vi "WAMP to LV error.vi"(8 "error in (no error)":errorcluster, 9 "Details Index":u32=3, 11 "WAMP Message":T2 {"Message Codes" items=["HELLO"=1, "WELCOME"=2, "ABORT"=3, "GOODBYE"=6, "ERROR"=8, "PUBLISH"=16, "PUBLISHED"=17, "SUBSCRIBE"=32, "SUBSCRIBED"=33, "UNSUBSCRIBE"=34, "UNSUBSCRIBED"=35, "EVENT"=36, "CALL"=48, "RESULT"=59, "REGISTER"=64, "REGISTERED"=65, "UNREGISTER"=66, "UNREGISTERED"=67, "INVOCATION"=68, "YIELD"=70]}) -> (0 "error out":errorcluster, 1 "Cluster":T1={"Details"="{}", "ArgumentKw Payload"="{}", "Error?"=FALSE, "Error URI"="", "Arguments Payload"=[]})   [LabVIEW 2020, in "wamplv.lvlib" / "WAMP Client.lvclass"]
uses:
  <userlib>/wamplv/WAMP Client/WAMP Client.lvclass
  <userlib>/wamplv/WAMP Client/TypeDef/WAMP Received Message.ctl
  <userlib>/wamplv/WAMP Message Codes.ctl
  <userlib>/wamplv/WAMP Client/TypeDef/WAMP Error Payload.ctl
  <vilib>/Utility/error.llb/Error Cluster From Error Code.vi
  <vilib>/ErrorRing/Error Ring.xnode
  <vilib>/JDP Science/JSONtext/JSONtext.lvlib
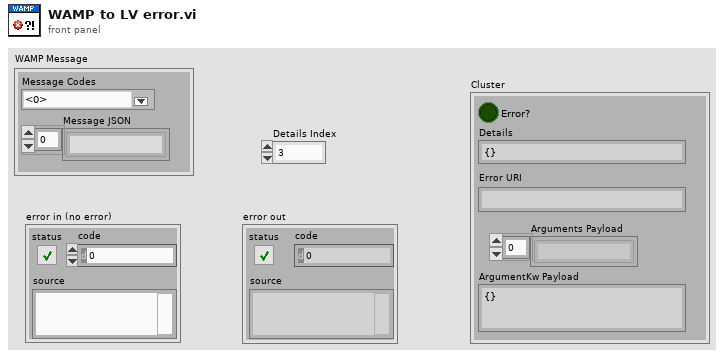
[diagram p1: front panel]
types:
  T1 = typedef "wamplv.lvlib/WAMP Client.lvclass/WAMP Error Payload.ctl" = cluster{"Details":string, "ArgumentKw Payload":string, "Error?":bool, "Error URI":string, "Arguments Payload":string[]}
  T2 = typedef "wamplv.lvlib/WAMP Client.lvclass/WAMP Received Message.ctl" = cluster{"Message JSON":string[], "Message Codes":T3}
  T3 = typedef "wamplv.lvlib/WAMP Client.lvclass/WAMP Message Codes.ctl" = u16
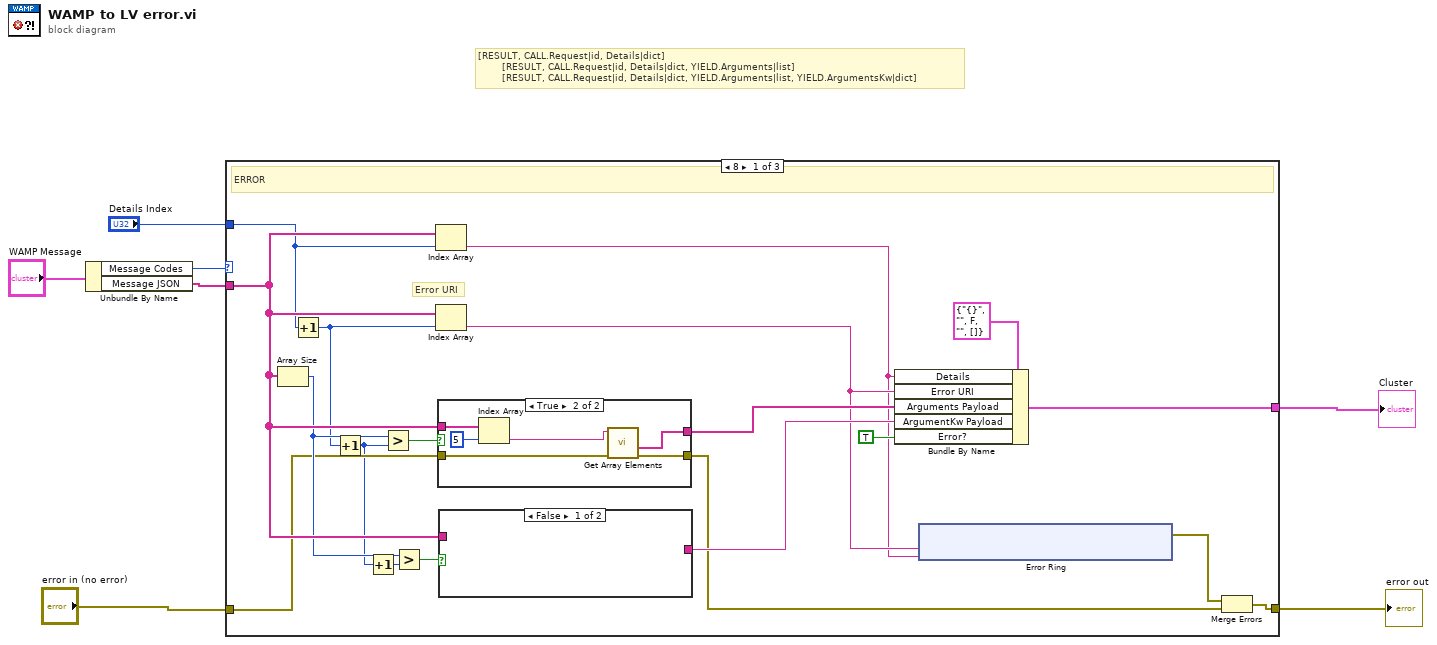
[diagram p0: block diagram]
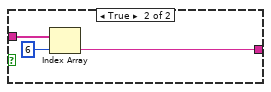
[diagram p2: hidden frame]
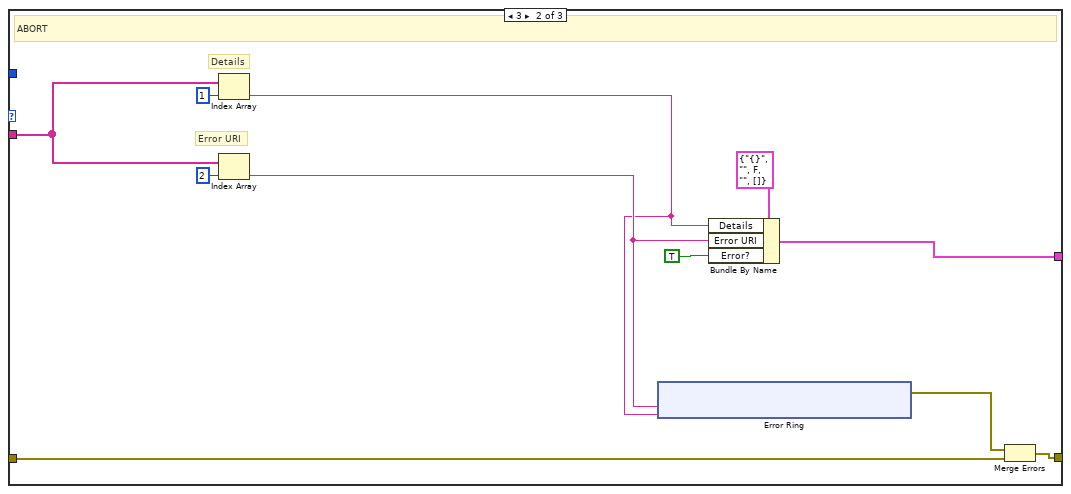
[diagram p4: hidden frame]
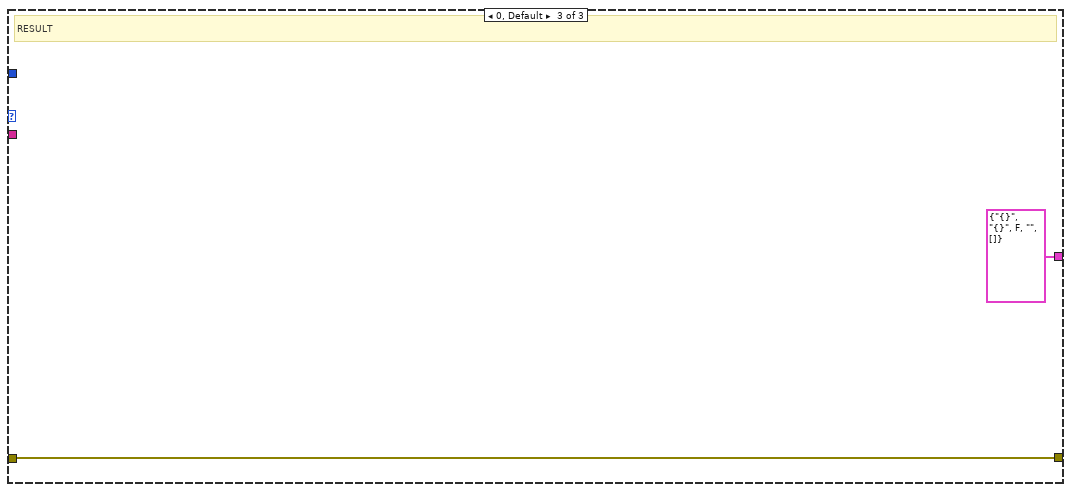
[diagram p5: hidden frame]
diagram:
  # "[RESULT, CALL.Request|id, Details|dict]\n        [RESULT, CALL.Request|id, Details|dict, YIELD.Arguments|list]\n        [RESULT, CALL.Request|id, Details|dict, YIELD.Arguments|list, YIELD.ArgumentsKw|dict]"
  n1 = Unbundle By Name("WAMP Message") -> ("Message Codes"=w5:T3, "Message JSON"=w4:string[])
  n2 = case shown="8" w5 {
    tunnel: w4 -> [w25 w55 _]
    tunnel: "error in (no error)" -> [w22 w48 w65]
    tunnel: [w13 w49 w65] -> w3
    tunnel: [w18 w52 T1 {"Details"="{}", "ArgumentKw Payload"="{}", "Error?"=FALSE, "Error URI"="", "Arguments Payload"=[]} ("Cluster")] -> w1
    tunnel: "Details Index" -> [w12 _ _]
    frame 8 {
      # "Error URI"
      # "ERROR"
      n3 = Array Size(array=w25) -> (size(s)=w23:i32)
      n4 = Increment(x=w12) -> (x+1=w11:u32)
      n5 = Increment(x=w11) -> (x+1=w9:u32)
      n6 = Increment(x=w9) -> (x+1=w10:u32)
      n7 = Greater?(x=w23, y=w9) -> (0:w26:bool)
      n8 = Greater?(x=w23, y=w10) -> (0:w24:bool)
      n9 = Index Array(array=w25, index=w12) -> (element=w8:string)
      n10 = Index Array(array=w25, index=w11) -> (element=w16:string)
      n11 = case shown="True" w26 {
        tunnel: w25 -> [_ w43]
        tunnel: w22 -> [w38 w39]
        tunnel: [w38 w40] -> w15
        tunnel: [_ w41] -> w17
        frame False {
        }
        frame True {
          n12 = Index Array(array=w43, index=5) -> (element=w42:string)
          n13 = call <vilib>:"Get Array Elements.vi"("error in (no error)"=w39, "JSON"=w42) -> ("error out"=w40:errorcluster, "<JSON>"=w41:string[])  [unwired: 7 in, 1 out]
        }
      }
      n14 = case shown="False" w24 {
        tunnel: [_ w36] -> w19
        tunnel: w25 -> [_ w35]
        frame False {
        }
        frame True {
          n15 = Index Array(array=w35, index=6) -> (element=w36:string)
        }
      }
      n16 = Bundle By Name(cluster=T1 {"Details"="{}", "ArgumentKw Payload"="", "Error?"=FALSE, "Error URI"="", "Arguments Payload"=[]} ("Cluster"), "Details"=w8, "Error URI"=w16, "Arguments Payload"=w17, "ArgumentKw Payload"=w19, "Error?"=TRUE ("status")) -> (w18:T1)
      n17 = xnode "Error Ring"("parameter 0"=w16, "parameter 1"=w8) -> ("error out"=w14:errorcluster)
      n18 = Merge Errors(w14, w15) -> (w13:errorcluster)
    }
    frame 3 {
      # "Details"
      # "Error URI"
      # "ABORT"
      n19 = Index Array(array=w55, index=1) -> (element=w47:string)
      n20 = Index Array(array=w55, index=2) -> (element=w51:string)
      n21 = xnode "Error Ring"("parameter 0"=w51, "parameter 1"=w47) -> ("error out"=w50:errorcluster)
      n22 = Bundle By Name(cluster=T1 {"Details"="{}", "ArgumentKw Payload"="", "Error?"=FALSE, "Error URI"="", "Arguments Payload"=[]} ("Cluster"), "Details"=w47, "Error URI"=w51, "Error?"=TRUE ("status")) -> (w52:T1)
      n23 = Merge Errors(w50, w48) -> (w49:errorcluster)
    }
    frame 0, Default {
      # "RESULT"
    }
  }
  "error out" <- w3
  "Cluster" <- w1
